vi "Host main.vi"() -> ()   [LabVIEW 2021]
panel:
  in  "Velocity Damping":dbl
  in  "Motors Enable":bool[](array[boolean])=[FALSE, FALSE, FALSE]
  in  "Tension Control":bool
  in  "OK Button":bool
  in  "Virtual Spring":dbl[](array[numeric])=[0.0, 0.0]
  in  "Path Radius":dbl(slide) scale=0.0..80.0
  in  "Record?":bool
  out "Tension":T1(graph)={"Numeric 4"=8.186601447964376, "Numeric 4"=8.30924819212997, "Numeric 4"=6.081676965828881, 20.263157894736842, 20.263157894736842, 20.263157894736842}
  in  "Lock":bool=TRUE
  in  "Simulation On":bool
  in  "ROS2 On":bool
  out "Robot Env":cluster{dbl[], dbl[]}[](graph)=[{[-2.0, 2.0, 0.0], [-2.0, -2.0, 2.0]}, {[0.0, 0.0, 0.0, 0.0, 0.0, 0.0, 0.0, 0.0, 0.0, -0.0, -0.0, -0.0, -0.0, -0.0, -0.0, -0.0, -0.0, -0.0, -0.0, -0.0, -0.0, -0.0, -0.0, -0.0, -0.0, 0.0, 0.0, 0.0, 0.0, 0.0, 0.0, 0.0], [0.0, 0.0, 0.0, 0.0, 0.0, 0.0, 0.0, 0.0, 0.0, 0.0, 0.0, 0.0, 0.0, 0.0, 0.0, 0.0, 0.0, -0.0, -0.0, -0.0, -0.0, -0.0, -0.0, -0.0, -0.0, -0.0, -0.0, -0.0, -0.0, -0.0, -0.0, -0.0]}, {[0.0], [-0.0]}, {[0.0], [0.0]}]
  in  "Manual Control":dbl[](array[slide])=[20.263157894736842, 20.263157894736842, 20.263157894736842] scale=0.0..50.0
  in  "Manual Control":bool=TRUE
  in  "Host Stop":bool
  # "Simulate"
  # "Message"
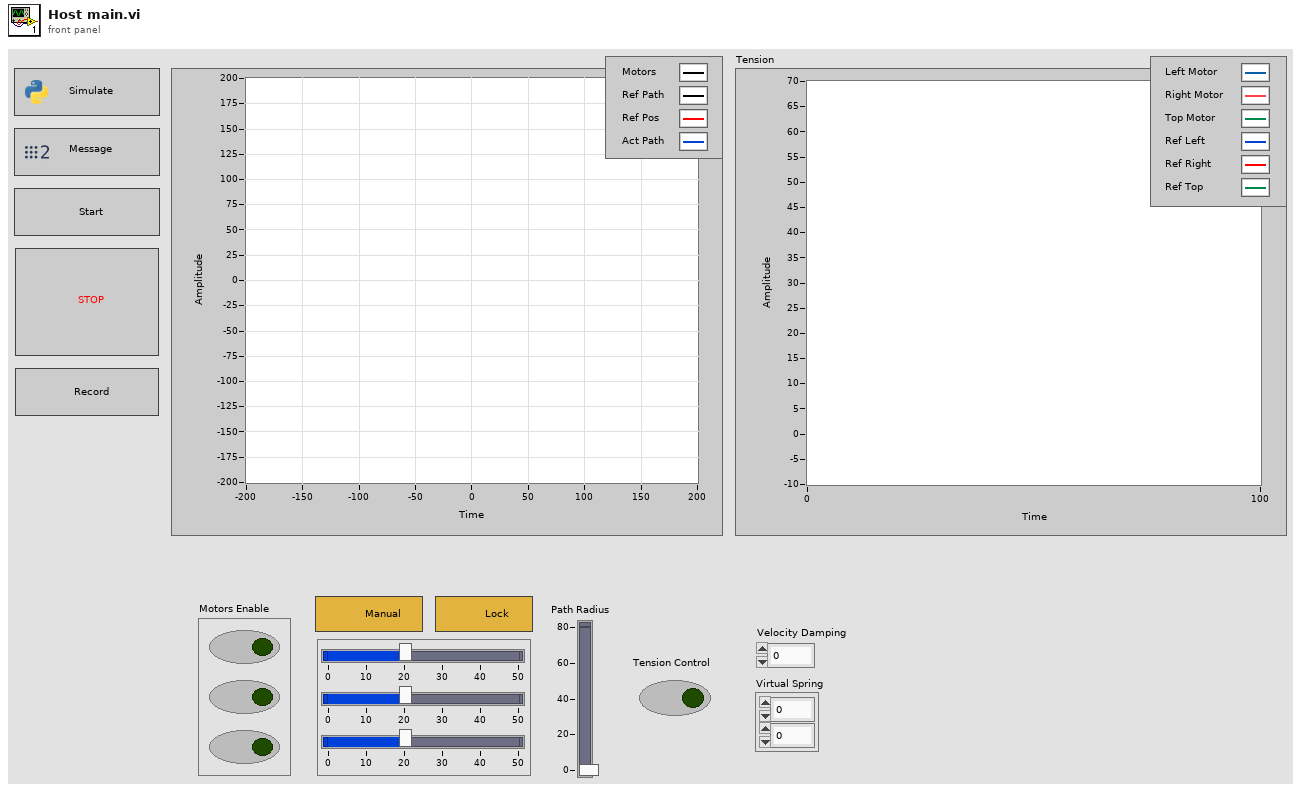
[diagram p1: front panel]
types:
  T1 = cluster{"Numeric 4":dbl, "Numeric 4":dbl, "Numeric 4":dbl, dbl, dbl, dbl}
  T2 = enum16{"open", "open or create", "create or replace", "create", "open (read-only)"}
  T3 = cluster{"Filtered x":dbl, "Filtered x":dbl, "Filtered x":dbl, dbl, dbl, dbl}
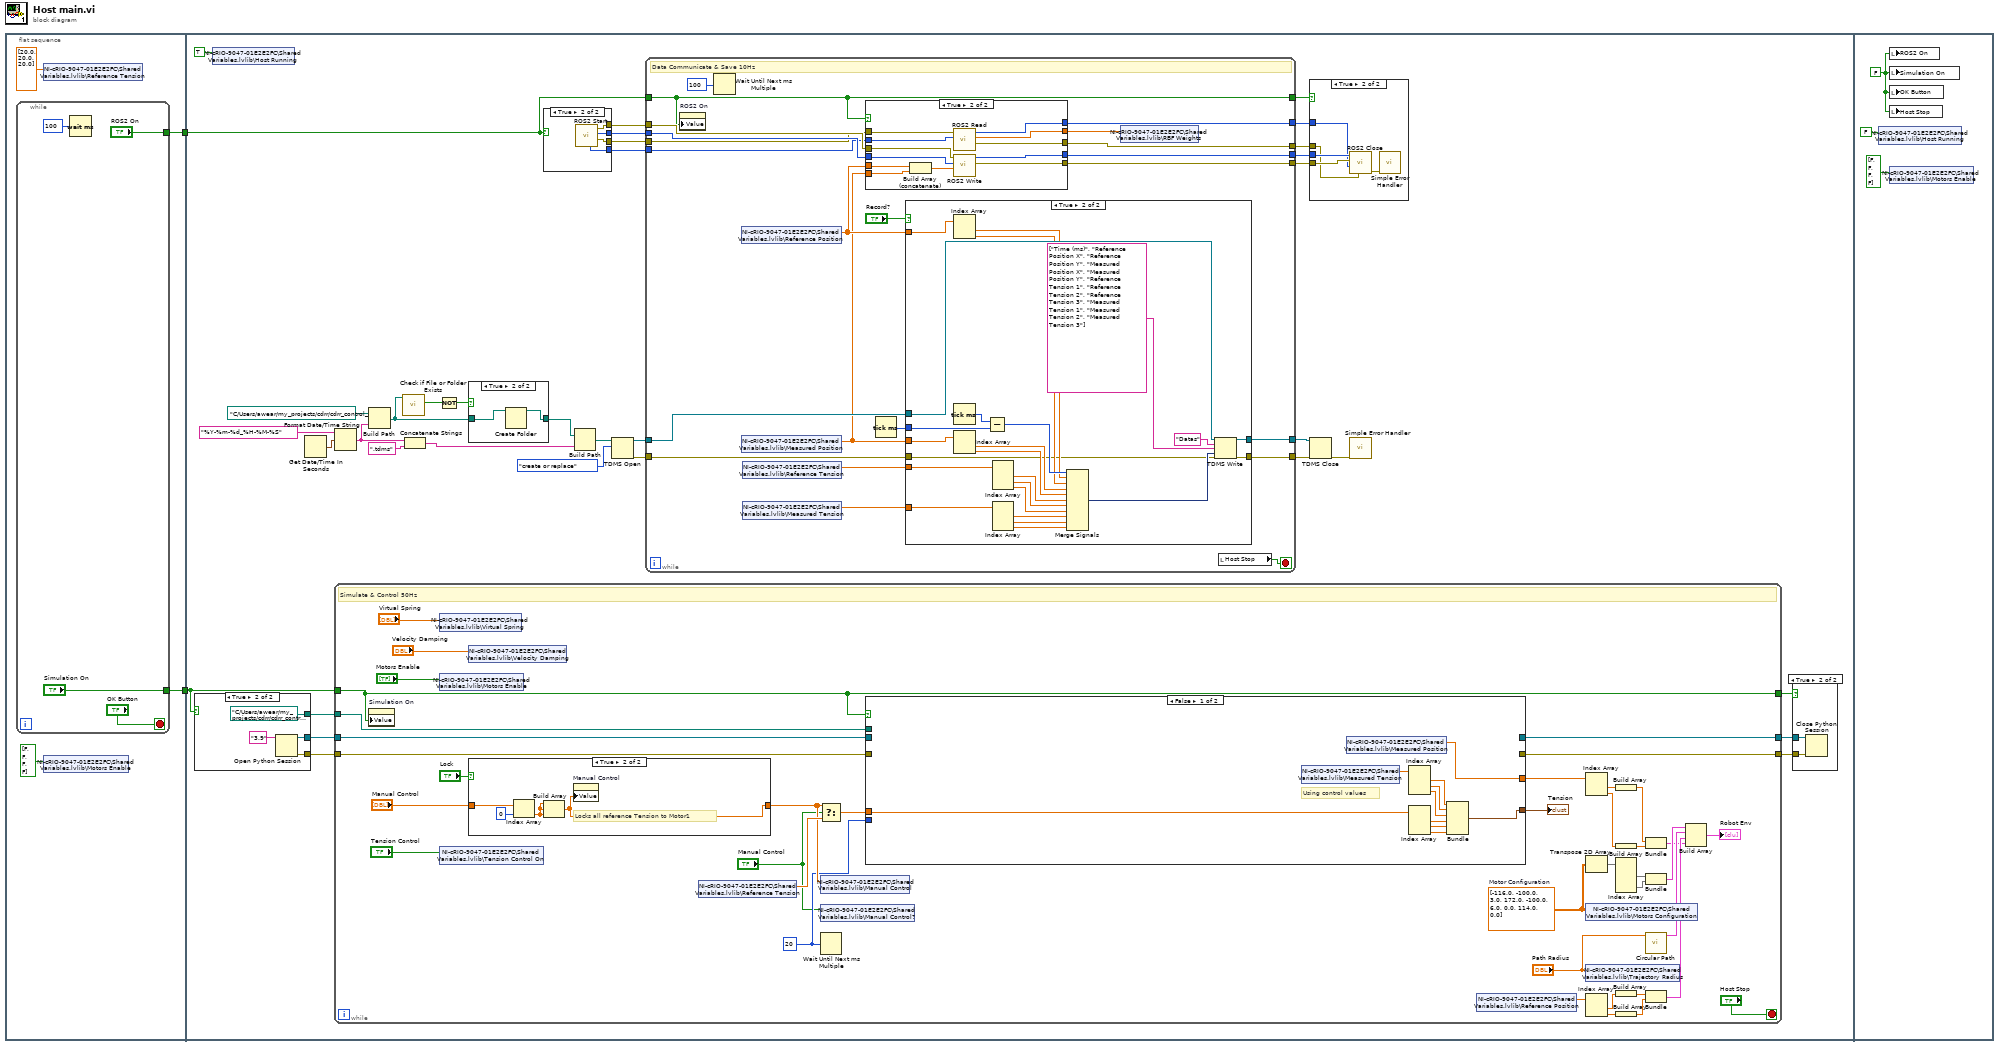
[diagram p0: block diagram]
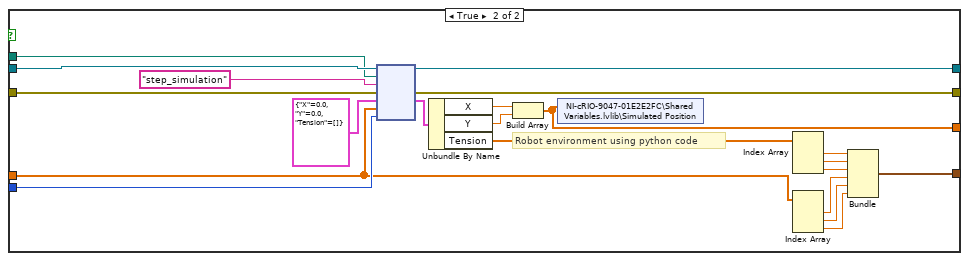
[diagram p8: hidden frame]
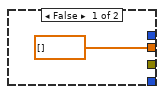
[diagram p9: hidden frame]
diagram:
  n1 = flat-sequence {
    tunnel: [w6] -> w2
    tunnel: [w5] -> w1
    tunnel: w2 -> [w27]
    tunnel: w1 -> [w26]
    frame #0 {
      n2 = while {
        tunnel: ["ROS2 On"] -> w6
        tunnel: ["Simulation On"] -> w5
        stop <- "OK Button" stop-if-true
        n3 = Wait (ms)(milliseconds to wait=u32 100 ("Period 2")) -> ()  [unwired: 1 out]
      }
      n4 = shared-variable "NI-cRIO-9047-01E2E2FC\\Shared Variables.lvlib\\Reference Tension"(dbl[] [20.0, 20.0, 20.0] ("Reference Tension")) -> ()  [unwired: 1 in, 1 out]
      n5 = shared-variable "NI-cRIO-9047-01E2E2FC\\Shared Variables.lvlib\\Motors Enable"(bool[] [FALSE, FALSE, FALSE, FALSE] ("Motors Enable")) -> ()  [unwired: 1 in, 1 out]
    }
    frame #1 {
      n6 = case shown="True" w26 {
        tunnel: [_ path "C:/Users/awear/my_projects/cdrr/cdrr_control_labview/Host PC/robot_env.py" ("module path")] -> w45
        tunnel: [_ w61] -> w44
        tunnel: [_ w60] -> w43
        frame False {
        }
        frame True {
          n7 = Open Python Session(python version="3.9" ("Python version")) -> (session out=w61:refnum<k35>, error out=w60:errorcluster)  [unwired: 2 in]
        }
      }
      n8 = shared-variable "NI-cRIO-9047-01E2E2FC\\Shared Variables.lvlib\\Host Running"(TRUE) -> ()  [unwired: 1 in, 1 out]
      n9 = Get Date/Time In Seconds() -> (seconds since 1Jan1904=w21:timestamp)
      n10 = Format Date/Time String(time format string (%c)="%Y-%m-%d_%H-%M-%S", seconds (now)=w21) -> (date/time string=w15:string)  [unwired: 1 in]
      n11 = while {
        tunnel: w44 -> [w99]
        tunnel: [w102] -> w24
        tunnel: w43 -> [w101]
        tunnel: [w100] -> w23
        tunnel: w45 -> [w98]
        tunnel: w26 -> [w73]
        tunnel: [w73] -> w25
        stop <- "Host Stop" stop-if-true
        w77 = dbl[][] [[-116.0, -100.0, 3.0], [172.0, -100.0, 6.0], [0.0, 114.0, 0.0]]  # Motor Configuration
        w81 = u32 20 ("Period 2")
        # "Simulate & Control 50Hz"
        n12 = property on="Simulation On" class="Bool (strict)"("Value"=w73) -> ()  [unwired: 2 in, 2 out]
        n13 = shared-variable "NI-cRIO-9047-01E2E2FC\\Shared Variables.lvlib\\Virtual Spring"("Virtual Spring") -> ()  [unwired: 1 in, 1 out]
        n14 = shared-variable "NI-cRIO-9047-01E2E2FC\\Shared Variables.lvlib\\Motors Enable"("Motors Enable") -> ()  [unwired: 1 in, 1 out]
        n15 = shared-variable "NI-cRIO-9047-01E2E2FC\\Shared Variables.lvlib\\Tension Control On"("Tension Control") -> ()  [unwired: 1 in, 1 out]
        n16 = shared-variable "NI-cRIO-9047-01E2E2FC\\Shared Variables.lvlib\\Velocity Damping"("Velocity Damping") -> ()  [unwired: 1 in, 1 out]
        n17 = case shown="True" "Lock" {
          tunnel: [w103 w104] -> w92
          tunnel: "Manual Control" -> [w103 w105]
          frame False {
          }
          frame True {
            # "Locks all reference Tension to Motor1"
            n18 = Index Array(array=w105, index=0) -> (element=w106:dbl)
            n19 = Build Array(w106, w106, w106) -> (w104:dbl[])
            n20 = property on="Manual Control" class="Arr (strict)"("Value"=w104) -> ()  [unwired: 2 in, 2 out]
          }
        }
        n21 = shared-variable "NI-cRIO-9047-01E2E2FC\\Shared Variables.lvlib\\Reference Tension"() -> (w95:dbl[])  [unwired: 1 in, 1 out]
        n22 = Select(t=w92, s="Manual Control", f=w95) -> (s? t:f=w94:dbl[])
        n23 = shared-variable "NI-cRIO-9047-01E2E2FC\\Shared Variables.lvlib\\Manual Control"(w92) -> ()  [unwired: 1 in, 1 out]
        n24 = shared-variable "NI-cRIO-9047-01E2E2FC\\Shared Variables.lvlib\\Manual Control?"("Manual Control") -> ()  [unwired: 1 in, 1 out]
        n25 = Wait Until Next ms Multiple(millisecond multiple=w81) -> ()  [unwired: 1 out]
        n26 = case shown="False" w73 {
          tunnel: [_ w137] -> w102
          tunnel: w101 -> [_ w136]
          tunnel: [_ w135] -> w100
          tunnel: w99 -> [_ w134]
          tunnel: w98 -> [_ w133]
          tunnel: w94 -> [w112 w121]
          tunnel: w81 -> [_ w131]
          tunnel: [w108 w123] -> w82
          tunnel: [w113 w122] -> w74
          frame False {
            # "Using control values"
            n27 = shared-variable "NI-cRIO-9047-01E2E2FC\\Shared Variables.lvlib\\Measured Tension"() -> (w114:dbl[])  [unwired: 1 in, 1 out]
            n28 = shared-variable "NI-cRIO-9047-01E2E2FC\\Shared Variables.lvlib\\Measured Position"() -> (w108:dbl[])  [unwired: 1 in, 1 out]
            n29 = Index Array(array=w114) -> (element #1=w117:dbl, element #2=w116:dbl, element #3=w115:dbl)  [unwired: 3 in]
            n30 = Index Array(array=w112) -> (element #1=w111:dbl, element #2=w110:dbl, element #3=w109:dbl)  [unwired: 3 in]
            n31 = Bundle("Filtered x"=w117, "Filtered x"=w116, "Filtered x"=w115, w111, w110, w109) -> (w113:T3)  [unwired: 1 in]
          }
          frame True {
            # "Robot environment using python code"
            n32 = node(w134, w133, "step_simulation" ("function name"), w136, cluster{"X":dbl, "Y":dbl, "Tension":dbl[]} {"X"=0.0, "Y"=0.0, "Tension"=[]} ("return value"), w121, w131) -> (w137:refnum<k35>, w135:errorcluster, w132:cluster{"X":dbl, "Y":dbl, "Tension":dbl[]})  [unwired: 2 in, 2 out]
            n33 = Unbundle By Name(w132) -> ("X"=w125:dbl, "Y"=w124:dbl, "Tension"=w126:dbl[])
            n34 = Build Array(w125, w124) -> (w123:dbl[])
            n35 = shared-variable "NI-cRIO-9047-01E2E2FC\\Shared Variables.lvlib\\Simulated Position"(w123) -> ()  [unwired: 1 in, 1 out]
            n36 = Index Array(array=w126) -> (element #1=w129:dbl, element #2=w128:dbl, element #3=w127:dbl)  [unwired: 3 in]
            n37 = Index Array(array=w121) -> (element #1=w120:dbl, element #2=w119:dbl, element #3=w118:dbl)  [unwired: 3 in]
            n38 = Bundle("Numeric 4"=w129, "Numeric 4"=w128, "Numeric 4"=w127, w120, w119, w118) -> (w122:T1)  [unwired: 1 in]
          }
        }
        "Tension" <- w74
        n39 = shared-variable "NI-cRIO-9047-01E2E2FC\\Shared Variables.lvlib\\Reference Position"() -> (w91:dbl[])  [unwired: 1 in, 1 out]
        n40 = Index Array(array=w82) -> (element #1=w86:dbl, element #2=w85:dbl)  [unwired: 2 in]
        n41 = Transpose 2D Array(2D array=w77) -> (transposed array=w80:dbl[][])
        n42 = shared-variable "NI-cRIO-9047-01E2E2FC\\Shared Variables.lvlib\\Motors Configuration"(w77) -> ()  [unwired: 1 in, 1 out]
        n43 = shared-variable "NI-cRIO-9047-01E2E2FC\\Shared Variables.lvlib\\Trajectory Radius"("Path Radius") -> ()  [unwired: 1 in, 1 out]
        n44 = Index Array(array=w91) -> (element #1=w90:dbl, element #2=w89:dbl)  [unwired: 2 in]
        n45 = Build Array(w86) -> (w84:dbl[])
        n46 = Build Array(w85) -> (w83:dbl[])
        n47 = Index Array(array=w80) -> (element #1=w79:dbl[], element #2=w78:dbl[])  [unwired: 4 in]
        n48 = Build Array(w90) -> (w88:dbl[])
        n49 = Build Array(w89) -> (w87:dbl[])
        n50 = Bundle(w84, w83) -> (w68:cluster{dbl[], dbl[]})  [unwired: 1 in]
        n51 = Bundle(w79, w78) -> (w71:cluster{dbl[], dbl[]})  [unwired: 1 in]
        n52 = call "Circular Path.vi"("Trajectory Radius"="Path Radius") -> ("Circular Path"=w70:cluster{dbl[], dbl[]})  [unwired: 10 in]
        n53 = Bundle(w88, w87) -> (w69:cluster{dbl[], dbl[]})  [unwired: 1 in]
        n54 = Build Array(w71, w70, w69, w68) -> (→"Robot Env":cluster{dbl[], dbl[]}[])
      }
      n55 = Build Path(base path=path "C:/Users/awear/my_projects/cdrr/cdrr_control_labview/data_save" ("file path"), name or relative path=w15) -> (appended path=w17:path)
      n56 = call <vilib>:"Check if File or Folder Exists.vi"("path"=w17) -> ("file or folder exists?"=w19:bool)  [unwired: 8 in, 2 out]
      n57 = Concatenate Strings(w15, ".tdms" ("string")) -> (w13:string)
      n58 = Not(x=w19) -> (.not. x?=w18:bool)
      n59 = case shown="True" w18 {
        tunnel: w17 -> [w46 w48]
        tunnel: [w46 w47] -> w16
        frame False {
        }
        frame True {
          n60 = Create Folder(path (use dialog)=w48) -> (created path=w47:path)  [unwired: 2 in, 2 out]
        }
      }
      n61 = case shown="True" w27 {
        tunnel: [_ w59] -> w38
        tunnel: [_ w58] -> w36
        tunnel: [_ w57] -> w34
        tunnel: [_ w56] -> w33
        frame False {
        }
        frame True {
          n62 = call "ROS2 Start.vi"() -> ("reader error"=w56:errorcluster[], "Writer"=w59:u64[], "writer error"=w58:errorcluster[], "Reader"=w57:u64[])  [unwired: 8 in]
        }
      }
      n63 = Build Path(base path=w16, name or relative path=w13) -> (appended path=w11:path)
      n64 = TDMS Open(10:T2."create or replace" ("operation (0:open)"), 11:w11) -> (0:w28:errorcluster, 3:w42:refnum<k34>)  [unwired: 5 in]
      n65 = while {
        tunnel: w42 -> [w160]
        tunnel: [w159] -> w41
        tunnel: w38 -> [w154]
        tunnel: [w153] -> w37
        tunnel: w36 -> [w152]
        tunnel: [w151] -> w35
        tunnel: w34 -> [w150]
        tunnel: w33 -> [w149]
        tunnel: [w148] -> w32
        tunnel: [w147] -> w31
        tunnel: w27 -> [w141]
        tunnel: [w141] -> w30
        tunnel: [w140] -> w29
        tunnel: w28 -> [w139]
        stop <- w156 stop-if-true
        # "Data Communicate & Save 10Hz"
        n66 = property on="ROS2 On" class="Bool (strict)"("Value"=w141) -> ()  [unwired: 2 in, 2 out]
        n67 = Wait Until Next ms Multiple(millisecond multiple=u32 100 ("Period 2")) -> ()  [unwired: 1 out]
        n68 = shared-variable "NI-cRIO-9047-01E2E2FC\\Shared Variables.lvlib\\Reference Position"() -> (w144:dbl[])  [unwired: 1 in, 1 out]
        n69 = shared-variable "NI-cRIO-9047-01E2E2FC\\Shared Variables.lvlib\\Measured Position"() -> (w143:dbl[])  [unwired: 1 in, 1 out]
        n70 = shared-variable "NI-cRIO-9047-01E2E2FC\\Shared Variables.lvlib\\Reference Tension"() -> (w146:dbl[])  [unwired: 1 in, 1 out]
        n71 = shared-variable "NI-cRIO-9047-01E2E2FC\\Shared Variables.lvlib\\Measured Tension"() -> (w145:dbl[])  [unwired: 1 in, 1 out]
        n72 = case shown="True" w141 {
          tunnel: w154 -> [_ w173]
          tunnel: [_ w172] -> w153
          tunnel: w152 -> [_ w171]
          tunnel: [_ w170] -> w151
          tunnel: w150 -> [_ w169]
          tunnel: w149 -> [_ w168]
          tunnel: [_ w167] -> w148
          tunnel: [_ w166] -> w147
          tunnel: w144 -> [_ w164]
          tunnel: w143 -> [_ w163]
          tunnel: [dbl[] [] w162] -> w142
          frame False {
          }
          frame True {
            n73 = Build Array (concatenate)(w164, w163) -> (w165:dbl[])
            n74 = call "ROS2 Read.vi"("DDS in"=w169, "error in"=w168) -> ("error out"=w167:errorcluster[], "Amplified Read"=w162:dbl[], "DDS out"=w166:u64[])  [unwired: 7 in]
            n75 = call "ROS2 Write.vi"("Data in"=w165, "DDS"=w173, "error in"=w171) -> ("error out"=w170:errorcluster[], "DDS out"=w172:u64[])  [unwired: 7 in]
          }
        }
        n76 = Tick Count (ms)() -> (millisecond timer value=w158:u32)
        n77 = case shown="True" "Record?" {
          tunnel: w160 -> [w175 w199]
          tunnel: [w174 w181] -> w140
          tunnel: [w175 w182] -> w159
          tunnel: w158 -> [_ w194]
          tunnel: w144 -> [_ w180]
          tunnel: w143 -> [_ w179]
          tunnel: w146 -> [_ w178]
          tunnel: w145 -> [_ w177]
          tunnel: w139 -> [w174 w176]
          frame False {
          }
          frame True {
            n78 = Index Array(array=w180) -> (element #1=w192:dbl, element #2=w191:dbl)  [unwired: 2 in]
            n79 = Tick Count (ms)() -> (millisecond timer value=w196:u32)
            n80 = Index Array(array=w179) -> (element #1=w190:dbl, element #2=w189:dbl)  [unwired: 2 in]
            n81 = Subtract(x=w196, y=w194) -> (x-y=w193:u32)
            n82 = Index Array(array=w178) -> (element #1=w188:dbl, element #2=w187:dbl, element #3=w186:dbl)  [unwired: 3 in]
            n83 = Index Array(array=w177) -> (element #1=w185:dbl, element #2=w184:dbl, element #3=w183:dbl)  [unwired: 3 in]
            n84 = Merge Signals(w193, w192, w191, w190, w189, w188, w187, w186, w185, w184, w183) -> (w197:dynamicdata)
            n85 = TDMS Write(0:w199, 5:"Datas" ("group name in (Untitled)"), 7:string[] ["Time (ms)", "Reference Position X", "Reference Position Y", "Measured Position X", "Measured Position Y", "Reference Tension 1", "Reference Tension 2", "Reference Tension 3", "Measured Tension 1", "Measured Tension 2", "Measured Tension 3"] ("channel name(s) in (Untitled)"), 9:w197, 11:w176) -> (4:w182:refnum<k34>, 15:w181:errorcluster)  [unwired: 1 in, 2 out]
          }
        }
        n86 = shared-variable "NI-cRIO-9047-01E2E2FC\\Shared Variables.lvlib\\RBF Weights"(w142) -> ()  [unwired: 1 in, 1 out]
        n87 = local read "Host Stop"() -> (w156:bool)
      }
      n88 = case shown="True" w30 {
        tunnel: w37 -> [_ w54]
        tunnel: w35 -> [_ w53]
        tunnel: w32 -> [_ w52]
        tunnel: w31 -> [_ w51]
        frame False {
        }
        frame True {
          n89 = call "ROS2 Close.vi"(6:"error in"=w52, 9:"DDS in"=w51, 10:"error in"=w53, 11:"DDS in"=w54) -> ("error out"=w55:errorcluster)  [unwired: 7 in]
          n90 = call <vilib>:"Simple Error Handler.vi"("error in (no error)"=w55) -> ()  [unwired: 4 in, 5 out]
        }
      }
      n91 = TDMS Close(8:w29, 11:w41) -> (0:w40:errorcluster)  [unwired: 1 out]
      n92 = call <vilib>:"Simple Error Handler.vi"("error in (no error)"=w40) -> ()  [unwired: 4 in, 5 out]
      n93 = case shown="True" w25 {
        tunnel: w24 -> [_ w50]
        tunnel: w23 -> [_ w49]
        frame False {
        }
        frame True {
          n94 = Close Python Session(session in=w50, error in=w49) -> ()  [unwired: 1 out]
        }
      }
    }
    frame #2 {
      w202 = FALSE ("ROS2 On")
      n95 = shared-variable "NI-cRIO-9047-01E2E2FC\\Shared Variables.lvlib\\Host Running"(FALSE) -> ()  [unwired: 1 in, 1 out]
      n96 = local write "ROS2 On"(w202) -> ()
      n97 = local write "Simulation On"(w202) -> ()
      n98 = local write "OK Button"(w202) -> ()
      n99 = local write "Host Stop"(w202) -> ()
      n100 = shared-variable "NI-cRIO-9047-01E2E2FC\\Shared Variables.lvlib\\Motors Enable"(bool[] [FALSE, FALSE, FALSE, FALSE] ("Motors Enable")) -> ()  [unwired: 1 in, 1 out]
    }
  }
